vi "Configure Engine Speed.vi"(8 "error in (no error)":errorcluster, 9 "NIVS.System Definition Root":refnum<k24>, 10 "VI Reference":refnum<vi>, 11 "Engine Speed Parameters in":T1) -> (0 "error out":errorcluster, 3 "Engine Speed Parameters out":T1)   [LabVIEW 2013]
doc: "Use this template to create a dialog box with event handling."
uses:
  NationalInstruments.VeriStand.SystemStorage
  Support/Engine Speed Parameters.ctl
  NationalInstruments.VeriStand.SystemStorageUI
  <vilib>/NI Veristand/UI Controls/Single Node Browser/NI_VS UI Single Node Browser.lvlib
panel:
  in  "Dial Max RPM":dbl
  in  "Make Current Values Default":bool
  in  "Bind to Two?":bool=TRUE
  in  "Desired Speed":refnum<k24>(container)
  out "PWM Config Tab":enum32{"One", "Two"}(tab)=enum."Two"
  in  "Show Fixed?":bool
  in  "Fixed Speed":refnum<k24>(container)
  in  "Right Pane":u32(colorbox)=16448250
  in  "Left Pane":u32(colorbox)=65532
  in  "Top Pane color":u32(colorbox)=15400704
  in  "Control Label":string
  in  "OK":bool
  in  "Cancel":bool
  # "Channel Bindings"
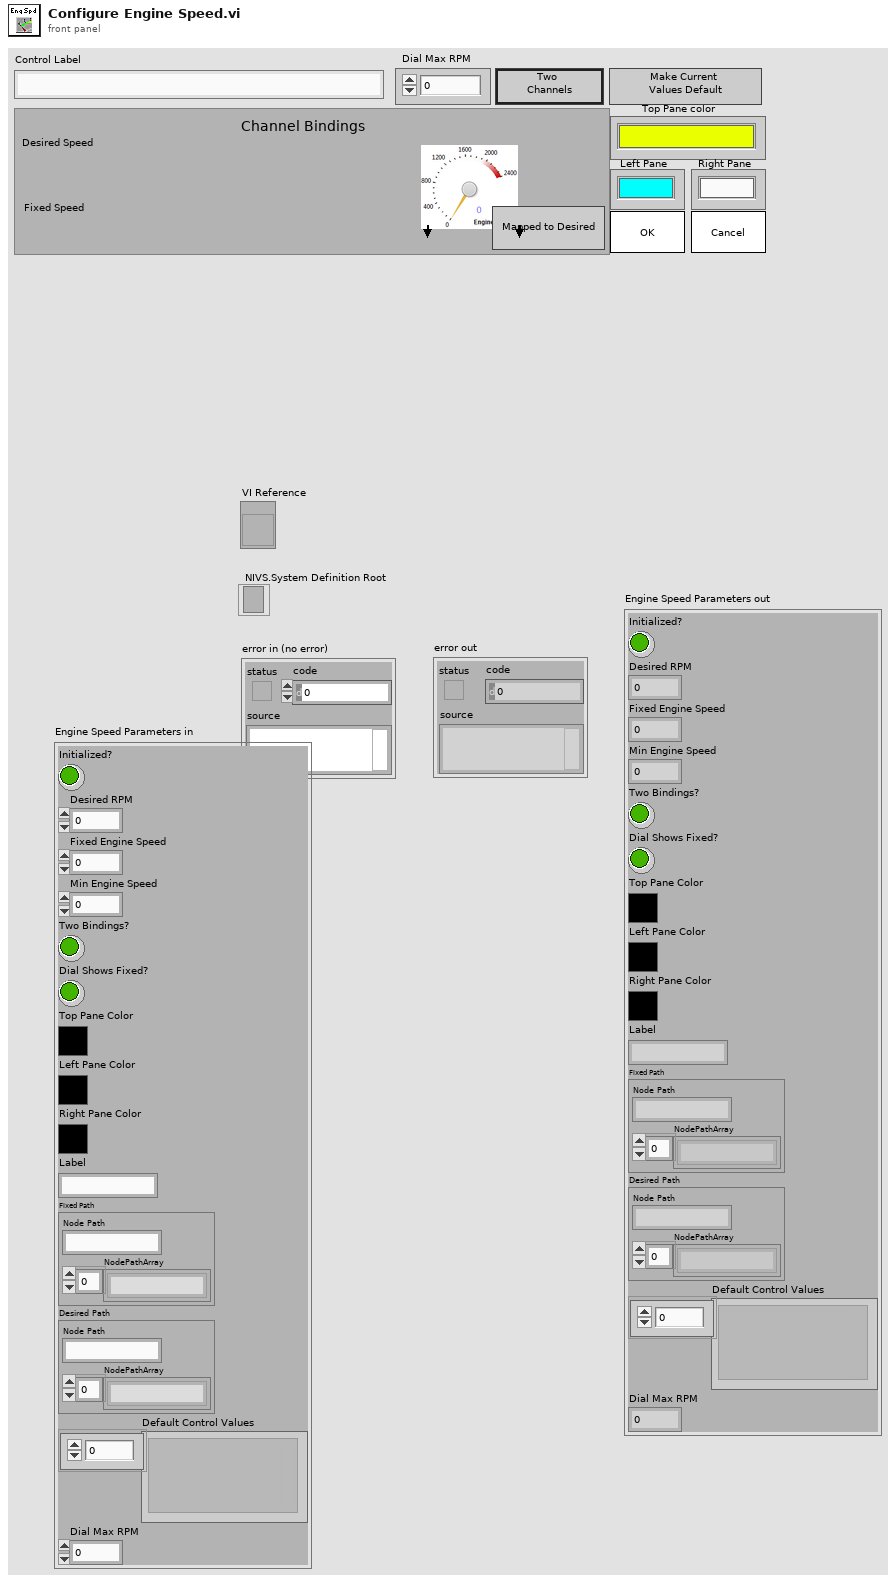
[diagram p1: front panel]
types:
  T1 = typedef "Engine Speed Parameters.ctl" = cluster{"Initialized?":bool, "Desired RPM":dbl, "Fixed Engine Speed":dbl, "Min Engine Speed":dbl, "Two Bindings? ":bool, "Dial Shows Fixed?":bool, "Top Pane Color":u32, "Left Pane Color":u32, "Right Pane Color":u32, "Label":string, "Fixed Path":cluster{"NodePathArray":string[], "Node Path":string}, "Desired Path":cluster{"NodePathArray":string[], "Node Path":string}, "Default Control Values":variant[], "Dial Max RPM":dbl}
  T2 = typedef "NI_VS UI Single Node Browser.lvlib/Callback Type.ctl" = cluster{"Net Callbacks":refnum<k27>[], "Event":refnum<user-event>}
  T3 = typedef "NI_VS UI Single Node Browser.lvlib/Node Ref.ctl" = refnum<k24>
  T4 = cluster{"NodePathArray":string[], "Node Path":string}
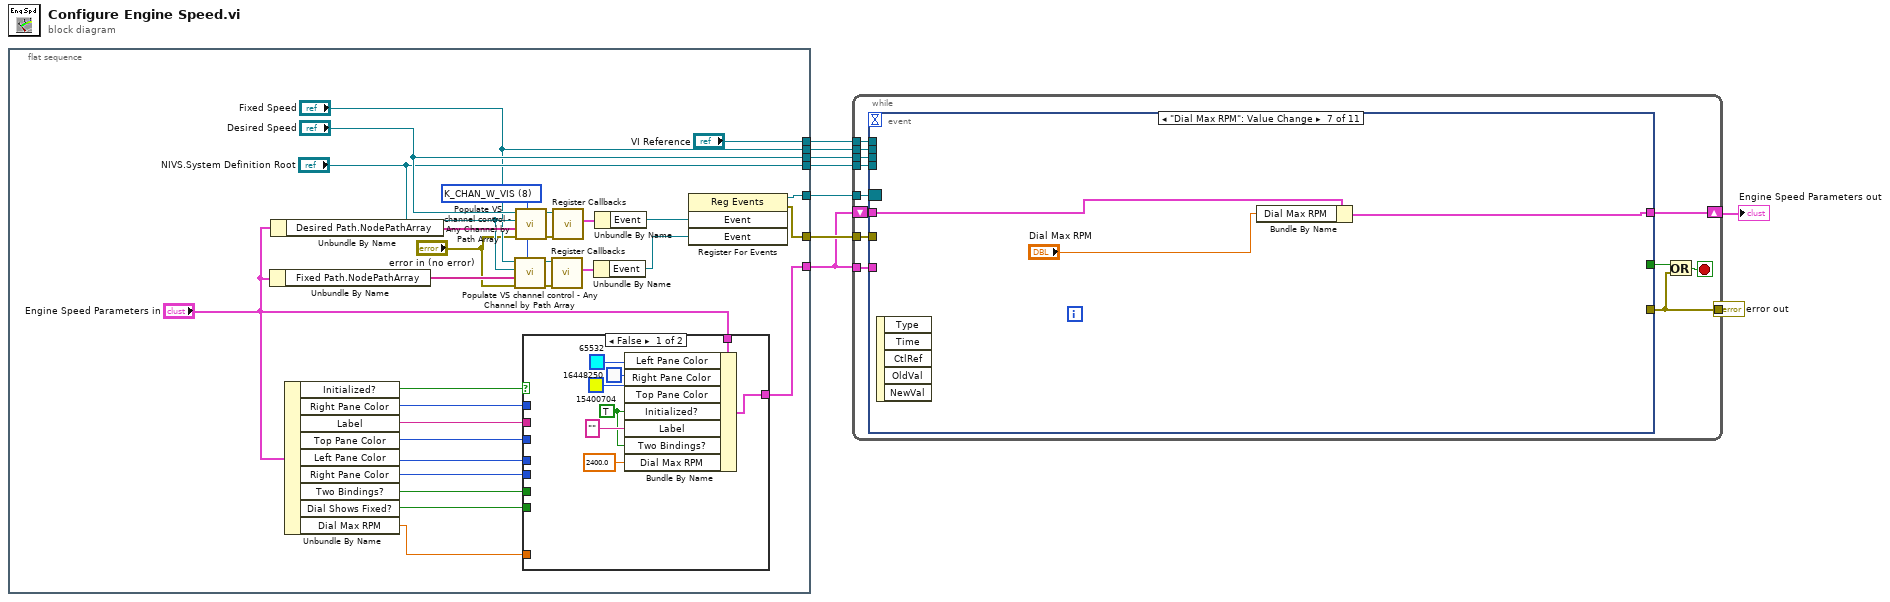
[diagram p0: block diagram]
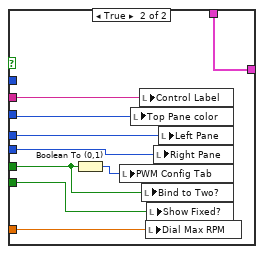
[diagram p2: hidden frame]
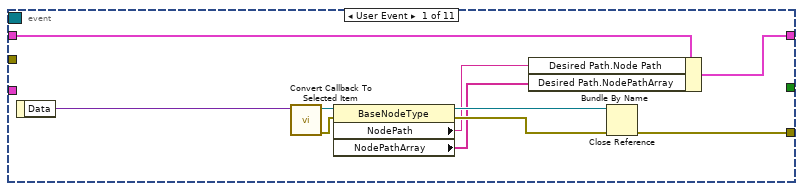
[diagram p3: hidden frame]
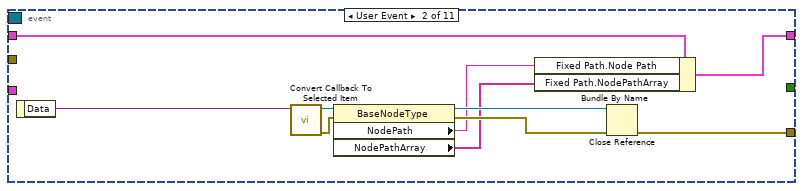
[diagram p4: hidden frame]
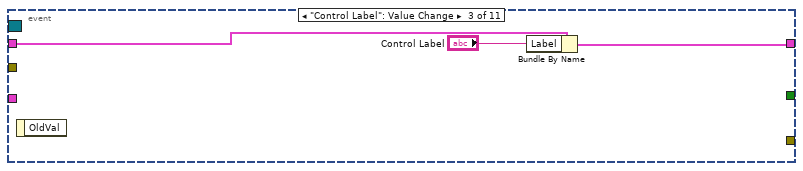
[diagram p5: hidden frame]
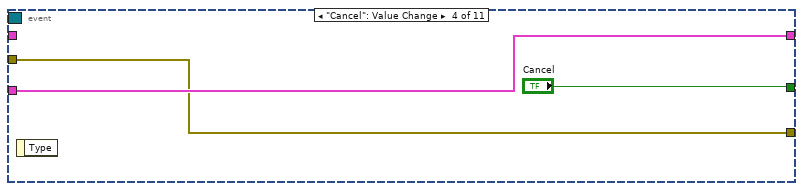
[diagram p6: hidden frame]
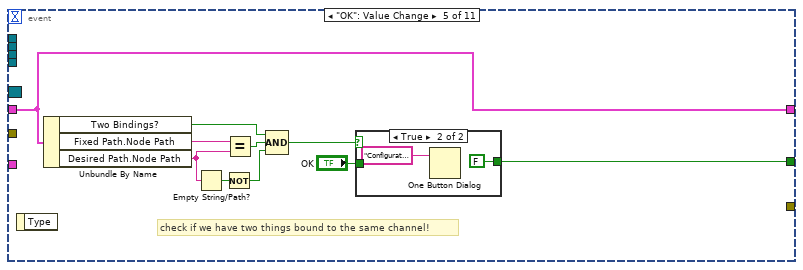
[diagram p7: hidden frame]
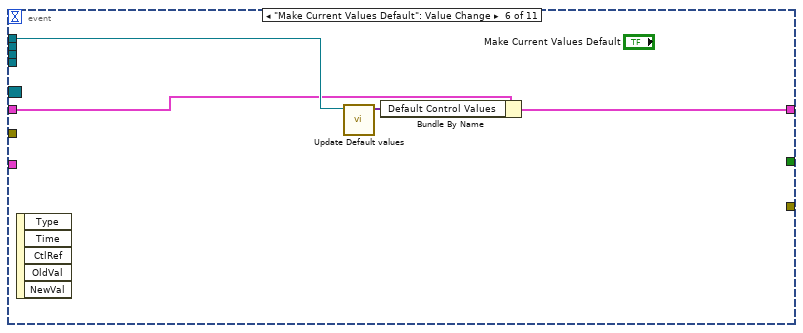
[diagram p9: hidden frame]
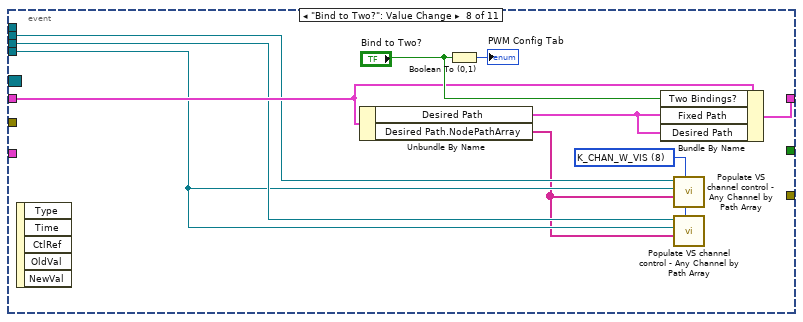
[diagram p10: hidden frame]
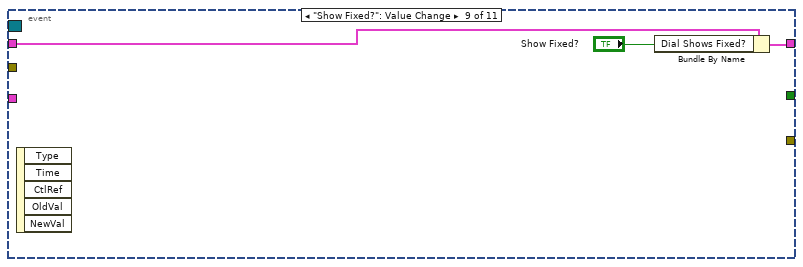
[diagram p11: hidden frame]
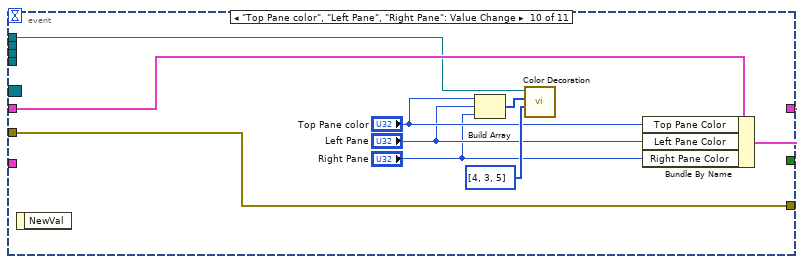
[diagram p12: hidden frame]
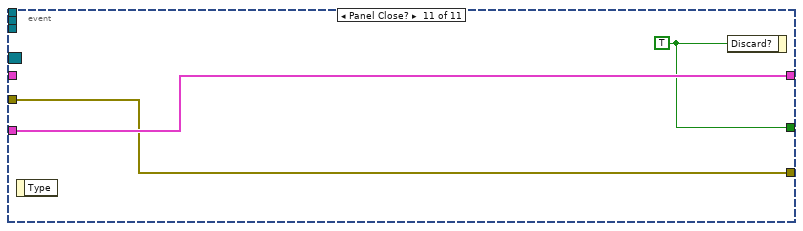
[diagram p13: hidden frame]
diagram:
  n1 = flat-sequence {
    tunnel: ["Desired Speed"] -> w8
    tunnel: ["NIVS.System Definition Root"] -> w7
    tunnel: [w28] -> w6
    tunnel: [w34] -> w1
    tunnel: ["VI Reference"] -> w5
    tunnel: [w27] -> w4
    tunnel: ["Fixed Speed"] -> w2
    frame #0 {
      w21 = u8 8 items=["K_CHAN_R", "K_CHAN_W", "K_CHAN_RW", "K_CHAN_VOLT", "K_CHAN_FAULT", "K_ALL", "K_CUSTOM", "K_CHAN_R_VIS", "K_CHAN_W_VIS", "K_CHAN_RW_VIS", "K_CHAN_VOLT_VIS", "K_CHAN_FAULT_VIS"] ("DisplayFilter")
      n2 = Unbundle By Name("Engine Speed Parameters in") -> ("Fixed Path.NodePathArray"=w18:string[])
      n3 = Unbundle By Name("Engine Speed Parameters in") -> ("Desired Path.NodePathArray"=w26:string[])
      n4 = Unbundle By Name("Engine Speed Parameters in") -> ("Initialized?"=w35:bool, "Right Pane Color"=w38:u32, "Label"=w37:string, "Top Pane Color"=w36:u32, "Left Pane Color"=w16:u32, "Right Pane Color"=w15:u32, "Two Bindings?"=w14:bool, "Dial Shows Fixed?"=w13:bool, "Dial Max RPM"=w10:dbl)
      n5 = call "Populate VS channel control - Any Channel by Path Array.vi"("DisplayFilter"=w21, "error in (no error)"="error in (no error)", "Path Array In"=w18, "NIVS.System Definition Root"="NIVS.System Definition Root", ".NET Refnum in"="Fixed Speed") -> ("error out"=w24:errorcluster, ".NET Refnum out"=w23:refnum<k24>)  [unwired: 5 in]
      n6 = call "Populate VS channel control - Any Channel by Path Array.vi"("DisplayFilter"=w21, "error in (no error)"="error in (no error)", "Path Array In"=w26, "NIVS.System Definition Root"="NIVS.System Definition Root", ".NET Refnum in"="Desired Speed") -> ("error out"=w29:errorcluster, ".NET Refnum out"=w30:refnum<k24>)  [unwired: 5 in]
      n7 = case shown="False" w35 {
        tunnel: w38 -> [_ _]
        tunnel: w37 -> [_ w55]
        tunnel: w36 -> [_ w54]
        tunnel: "Engine Speed Parameters in" -> [w46 w53]
        tunnel: [w45 w53] -> w34
        tunnel: w16 -> [_ w52]
        tunnel: w15 -> [_ w51]
        tunnel: w14 -> [_ w49]
        tunnel: w13 -> [_ w48]
        tunnel: w10 -> [_ w47]
        frame False {
          w40 = TRUE ("New?")
          n8 = Bundle By Name(cluster=w46, "Left Pane Color"=u32 65532, "Right Pane Color"=u32 16448250, "Top Pane Color"=u32 15400704, "Initialized?"=w40, "Label"="", "Two Bindings?"=w40, "Dial Max RPM"=2400.0) -> (w45:T1)
        }
        frame True {
          n9 = Boolean To (0,1)(Boolean=w49) -> (0, 1=w50:i16)
          n10 = local write "PWM Config Tab"(w50) -> ()
          n11 = local write "Top Pane color"(w54) -> ()
          n12 = local write "Control Label"(w55) -> ()
          n13 = local write "Bind to Two?"(w49) -> ()
          n14 = local write "Dial Max RPM"(w47) -> ()
          n15 = local write "Show Fixed?"(w48) -> ()
          n16 = local write "Right Pane"(w51) -> ()
          n17 = local write "Left Pane"(w52) -> ()
        }
      }
      n18 = call <vilib>:"Register Callbacks.vi"("error in (no error)"=w24, "Single Node Browser"=w23) -> ("Callbacks"=w22:T2)  [unwired: 7 in, 2 out]
      n19 = call <vilib>:"Register Callbacks.vi"("error in (no error)"=w29, "Single Node Browser"=w30) -> ("Callbacks"=w32:T2)  [unwired: 7 in, 2 out]
      n20 = Unbundle By Name(w22) -> ("Event"=w17:refnum<user-event>)
      n21 = Unbundle By Name(w32) -> ("Event"=w31:refnum<user-event>)
      n22 = register-events(w31, w17) -> (reference out=w27:refnum<event-registration>, error out=w28:errorcluster)  [unwired: 2 in]
    }
  }
  n23 = while {
    tunnel: [w57] -> w9
    shift-right: [w64] -> w3
    shift-left: w1 -> [w66]
    tunnel: w1 -> [w65]
    tunnel: w8 -> [w62]
    tunnel: w7 -> [w61]
    tunnel: w6 -> [w60]
    tunnel: w5 -> [w59]
    tunnel: w4 -> [w58]
    tunnel: w2 -> [w56]
    stop <- w63 stop-if-true
    n24 = event shown="[6] \"Dial Max RPM\": Value Change" {
      selector: w58 -> [_ _ _ _ _ _ _ _ _ _ _]
      dyn-events: _ -> [_ _ _ _ _ _ _ _ _ _ _]
      timeout: _ -> [_ _ _ _ _ _ _ _ _ _ _]
      tunnel: [_ _ _ "Cancel" w99 _ _ _ _ _ w137] -> w67
      tunnel: [w69 w79 _ w91 _ _ _ _ _ w133 w136] -> w57
      tunnel: w66 -> [w70 w80 w89 _ w95 w108 w113 w120 w126 w134 _]
      tunnel: w65 -> [_ _ _ w92 _ _ _ _ _ _ w138]
      tunnel: [w68 w78 w90 w92 w95 w109 w111 w121 w125 w135 w138] -> w64
      tunnel: w62 -> [_ _ _ _ _ _ _ w117 _ _ _]
      tunnel: w61 -> [_ _ _ _ _ _ _ w115 _ _ _]
      tunnel: w60 -> [_ _ _ w91 _ _ _ _ _ w133 w136]
      tunnel: w59 -> [_ _ _ _ _ w110 _ _ _ w131 _]
      tunnel: w56 -> [_ _ _ _ _ _ _ w118 _ _ _]
      event User Event {
        n25 = event-data() -> ("Data"=w71:variant)  [unwired: 1 in]
        n26 = call <vilib>:"Convert Callback To Selected Item.vi"("Data"=w71) -> ("error out"=w74:errorcluster, "Selected Item"=w77:T3)  [unwired: 9 in]
        n27 = property class="BaseNodeType"(reference=w77, error in=w74) -> (reference out=w76:T3, error out=w75:errorcluster, "NodePath"=w73:string, "NodePathArray"=w72:string[])
        n28 = Bundle By Name(cluster=w70, "Desired Path.Node Path"=w73, "Desired Path.NodePathArray"=w72) -> (w68:T1)
        n29 = Close Reference(reference=w76, error in (no error)=w75) -> (error out=w69:errorcluster)
      }
      event User Event {
        n30 = event-data() -> ("Data"=w81:variant)  [unwired: 1 in]
        n31 = call <vilib>:"Convert Callback To Selected Item.vi"("Data"=w81) -> ("error out"=w84:errorcluster, "Selected Item"=w87:T3)  [unwired: 9 in]
        n32 = property class="BaseNodeType"(reference=w87, error in=w84) -> (reference out=w86:T3, error out=w85:errorcluster, "NodePath"=w83:string, "NodePathArray"=w82:string[])
        n33 = Bundle By Name(cluster=w80, "Fixed Path.Node Path"=w83, "Fixed Path.NodePathArray"=w82) -> (w78:T1)
        n34 = Close Reference(reference=w86, error in (no error)=w85) -> (error out=w79:errorcluster)
      }
      event "Control Label": Value Change {
        n35 = event-data() -> ()  [unwired: 1 in, 1 out]
        n36 = Bundle By Name(cluster=w89, "Label"="Control Label") -> (w90:T1)
      }
      event "Cancel": Value Change {
        n37 = event-data() -> ()  [unwired: 1 in, 1 out]
      }
      event "OK": Value Change {
        # "check if we have two things bound to the same channel!"
        n38 = event-data() -> ()  [unwired: 1 in, 1 out]
        n39 = Unbundle By Name(w95) -> ("Two Bindings?"=w101:bool, "Fixed Path.Node Path"=w103:string, "Desired Path.Node Path"=w98:string)
        n40 = Empty String/Path?(string/path=w98) -> (empty?=w97:bool)
        n41 = Not(x=w97) -> (.not. x?=w96:bool)
        n42 = Equal?(x=w103, y=w98) -> (x = y?=w102:bool)
        n43 = Compound Arithmetic op=AND(w101, w102, w96) -> (w100:bool)
        n44 = case shown="True" w100 {
          tunnel: [w104 FALSE ("OK")] -> w99
          tunnel: "OK" -> [w104 _]
          frame False {
          }
          frame True {
            n45 = One Button Dialog(message="Configuration Invalid.\nTwo Channel Mode- please select two unique channels to bind." ("button name (\"OK\")")) -> ()  [unwired: 1 in, 1 out]
          }
        }
      }
      event "Make Current Values Default": Value Change {
        n46 = event-data() -> ()  [unwired: 1 in, 5 out]
        n47 = call "Update Default values.vi"("VI in"=w110) -> ("Default Values out"=w107:variant[])  [unwired: 10 in]
        n48 = Bundle By Name(cluster=w108, "Default Control Values"=w107) -> (w109:T1)
      }
      event "Dial Max RPM": Value Change {
        n49 = event-data() -> ()  [unwired: 1 in, 5 out]
        n50 = Bundle By Name(cluster=w113, "Dial Max RPM"="Dial Max RPM") -> (w111:T1)
      }
      event "Bind to Two?": Value Change {
        w116 = u8 8 items=["K_CHAN_R", "K_CHAN_W", "K_CHAN_RW", "K_CHAN_VOLT", "K_CHAN_FAULT", "K_ALL", "K_CUSTOM", "K_CHAN_R_VIS", "K_CHAN_W_VIS", "K_CHAN_RW_VIS", "K_CHAN_VOLT_VIS", "K_CHAN_FAULT_VIS"] ("DisplayFilter")
        n51 = event-data() -> ()  [unwired: 1 in, 5 out]
        n52 = Unbundle By Name(w120) -> ("Desired Path"=w119:T4, "Desired Path.NodePathArray"=w114:string[])
        n53 = Boolean To (0,1)(Boolean="Bind to Two?") -> (0, 1=→"PWM Config Tab":i16)
        n54 = Bundle By Name(cluster=w120, "Two Bindings?"="Bind to Two?", "Fixed Path"=w119, "Desired Path"=w119) -> (w121:T1)
        n55 = call "Populate VS channel control - Any Channel by Path Array.vi"("DisplayFilter"=w116, "Path Array In"=w114, "NIVS.System Definition Root"=w115, ".NET Refnum in"=w118) -> ()  [unwired: 6 in, 2 out]
        n56 = call "Populate VS channel control - Any Channel by Path Array.vi"("DisplayFilter"=w116, "Path Array In"=w114, "NIVS.System Definition Root"=w115, ".NET Refnum in"=w117) -> ()  [unwired: 6 in, 2 out]
      }
      event "Show Fixed?": Value Change {
        n57 = event-data() -> ()  [unwired: 1 in, 5 out]
        n58 = Bundle By Name(cluster=w126, "Dial Shows Fixed?"="Show Fixed?") -> (w125:T1)
      }
      event "Top Pane color", "Left Pane", "Right Pane": Value Change {
        n59 = event-data() -> ()  [unwired: 1 in, 1 out]
        n60 = Build Array("Top Pane color", "Left Pane", "Right Pane") -> (w132:u32[])
        n61 = call "Color Decoration.vi"("VI reference"=w131, "Color Array"=w132, "Index Array"=u32[] [4, 3, 5] ("Color Array")) -> ()  [unwired: 7 in, 1 out]
        n62 = Bundle By Name(cluster=w134, "Top Pane Color"="Top Pane color", "Left Pane Color"="Left Pane", "Right Pane Color"="Right Pane") -> (w135:T1)
      }
      event Panel Close? {
        w137 = TRUE ("Cancel")
        n63 = event-data() -> ()  [unwired: 1 in, 1 out]
        n64 = event-data("Discard?"=w137) -> ()  [unwired: 1 in, 1 out]
      }
    }
    n65 = Or(x=w67, y=w57) -> (x .or. y?=w63:bool)
  }
  "error out" <- w9
  "Engine Speed Parameters out" <- w3
